vi "TimeStrDismantle.vi"(1 "LogEvent":refnum<vi>, 2 "VCI_CAN_OBJ_R":T1) -> (0 "TimeCluster":T2)   [LabVIEW 2013]
uses:
  Log.ctl
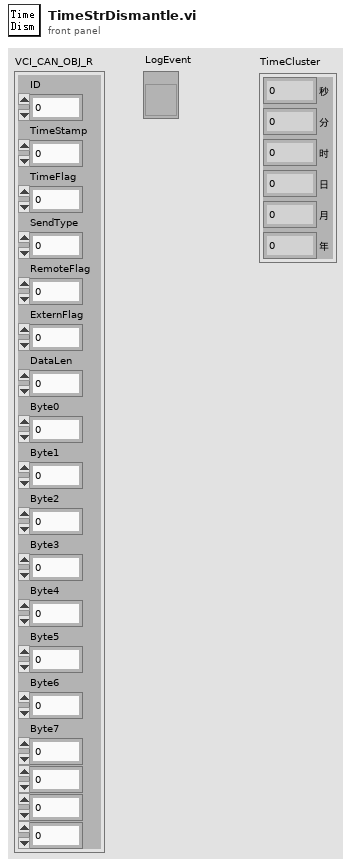
[diagram p1: front panel]
types:
  T1 = cluster{"ID":u32, "TimeStamp":u32, "TimeFlag":u8, "SendType":u8, "RemoteFlag":u8, "ExternFlag":u8, "DataLen":u8, "Byte0":u8, "Byte1":u8, "Byte2":u8, "Byte3":u8, "Byte4":u8, "Byte5":u8, "Byte6":u8, "Byte7":u8, u8, u8, u8}
  T2 = cluster{"秒":i32, "分":i32, "时":i32, "日":i32, "月":i32, "年":i32}
  T3 = typedef "Log.ctl" = cluster{"Event":string, "Value":variant}
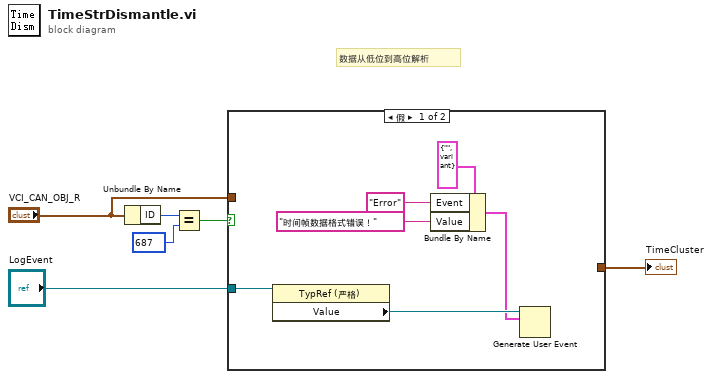
[diagram p0: block diagram]
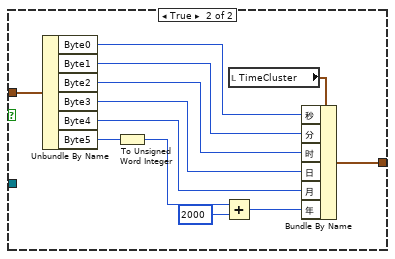
[diagram p2: hidden frame]
diagram:
  # "数据从低位到高位解析"
  n1 = Unbundle By Name("VCI_CAN_OBJ_R") -> ("ID"=w5:u32)
  n2 = Equal?(x=w5, y=u16 687) -> (x = y?=w3:bool)
  n3 = case shown="假" w3 {
    tunnel: [_ w21] -> w6
    tunnel: "VCI_CAN_OBJ_R" -> [_ w20]
    tunnel: "LogEvent" -> [w12 _]
    frame False {
      n4 = property class="TypRef (严格)"(reference=w12) -> ("Value"=w11:refnum<user-event>)  [unwired: 1 in, 2 out]
      n5 = Bundle By Name(cluster=T3 {"Event"="", "Value"=variant} ("Log"), "Event"="Error", "Value"="时间帧数据格式错误！" ("消息")) -> (w7:T3)
      n6 = Generate User Event(user event=w11, event data cluster=w7) -> ()  [unwired: 2 in, 2 out]
    }
    frame True {
      n7 = Unbundle By Name(w20) -> ("Byte0"=w19:u8, "Byte1"=w18:u8, "Byte2"=w17:u8, "Byte3"=w16:u8, "Byte4"=w15:u8, "Byte5"=w14:u8)
      n8 = To Unsigned Word Integer(number=w14) -> (unsigned 16bit integer=w13:u16)
      n9 = Add(x=w13, y=u16 2000) -> (x+y=w22:u16)
      n10 = local read "TimeCluster"() -> (w24:T2)
      n11 = Bundle By Name(cluster=w24, "秒"=w19, "分"=w18, "时"=w17, "日"=w16, "月"=w15, "年"=w22) -> (w21:T2)
    }
  }
  "TimeCluster" <- w6
